vi "readImageIfExists.vi"(8 "error in (no error)":errorcluster, 10 "appended path":path, 11 "Refnum in":T1) -> (0 "error out":errorcluster, 3 "Refnum out":T1)   [LabVIEW 2023]
uses:
  <vilib>/vision/Image Controls.llb/IMAQ Image.ctl
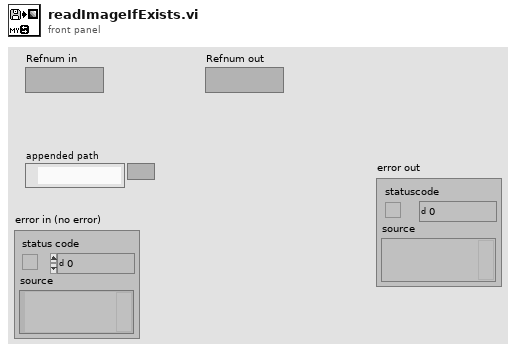
[diagram p1: front panel]
types:
  T1 = typedef "IMAQ Image.ctl" = refnum<image>
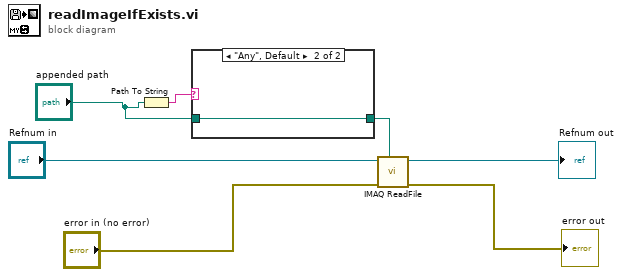
[diagram p0: block diagram]
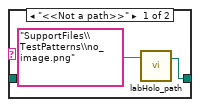
[diagram p2: hidden frame]
diagram:
  n1 = Path To String(path="appended path") -> (string=w2:string)
  n2 = case shown="\"Any\", Default" w2 {
    tunnel: [w8 w10] -> w5
    tunnel: "appended path" -> [_ w10]
    frame "<<Not a path>>" {
      n3 = call "labHolo_path.vi"("sub folder or file (str)"="SupportFiles\\TestPatterns\\no_image.png") -> ("labHolo path"=w8:path)  [unwired: 1 in, 1 out]
    }
    frame "Any", Default {
    }
  }
  n4 = call "IMAQ ReadFile"("File Path"=w5, "error in (no error)"="error in (no error)", "Image"="Refnum in") -> ("error out"=→"error out":errorcluster, "Image Out"=→"Refnum out":T1)  [unwired: 4 in, 3 out]
